vi "Untitled 4.vi"() -> ()   [LabVIEW 2014]
panel:
  in  "Function":enum16{"Init", "Get", "Set", ""}(ring)
  out "data_cluster_out":T1
  in  "data_cluster_in":T1
  out "switch_control_json":string
  out "switch_data_json":string
  out "train_control_json":string
  out "train_data_json":string
  out "train_data_out":T2
  out "switch_control_out":T3
  out "switch_data_out":T4
  out "train_control_out":T5
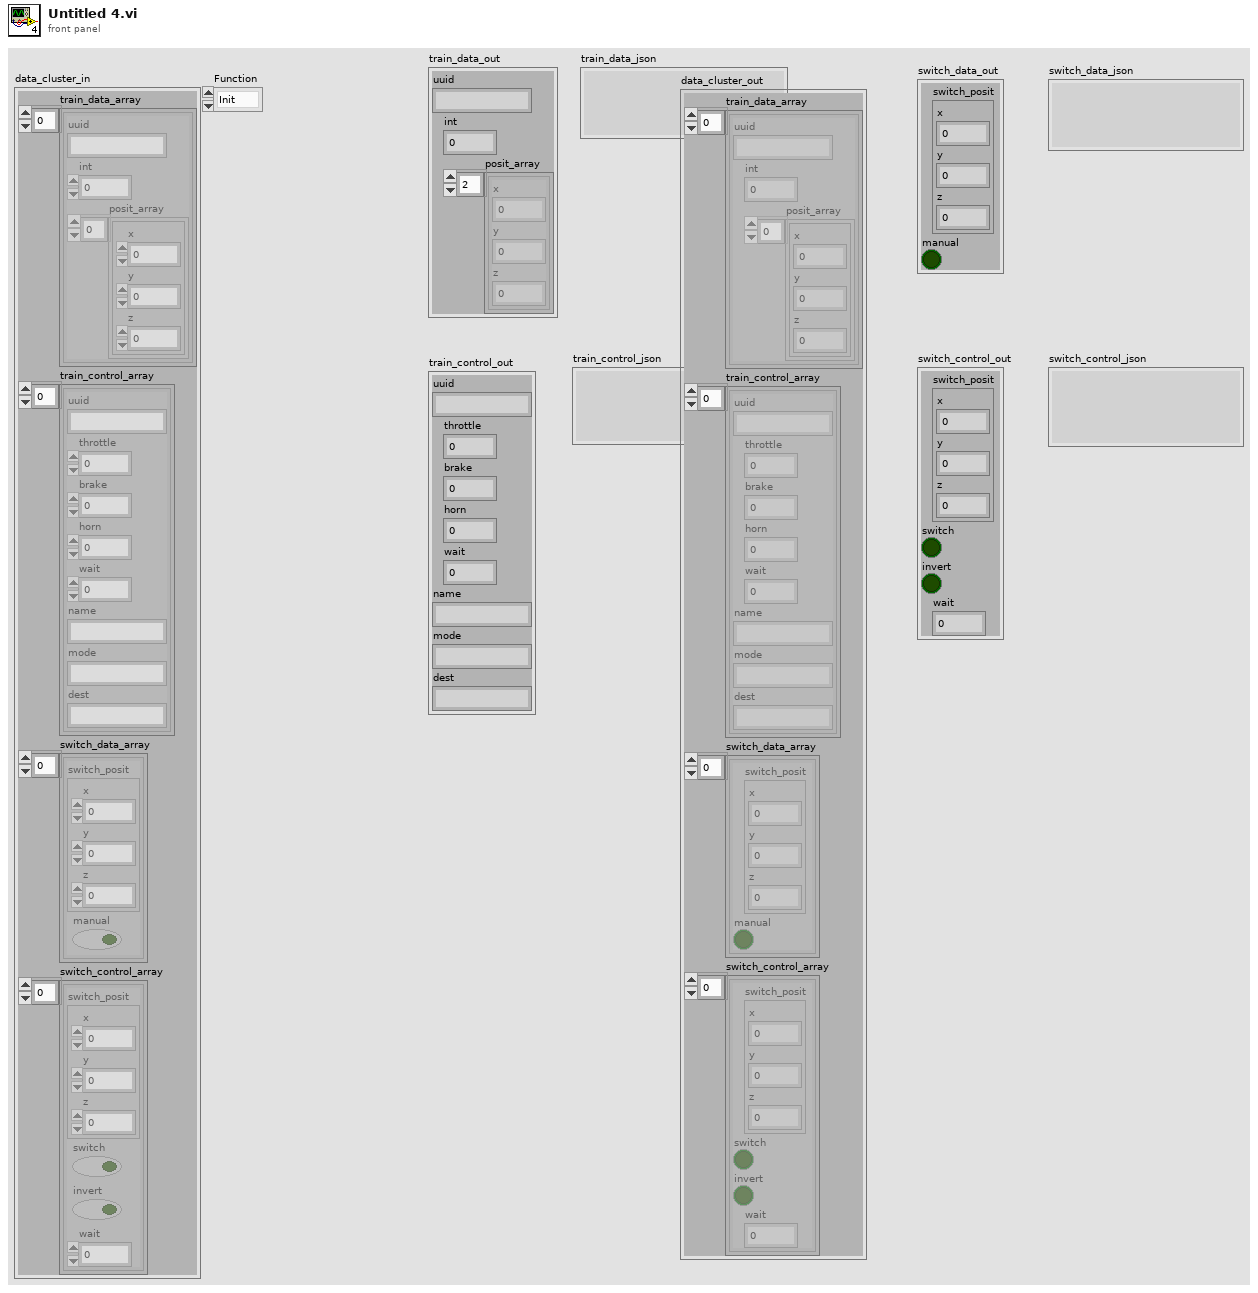
[diagram p1: front panel]
types:
  T1 = cluster{"train_data_array":cluster{"uuid":string, "int":i32, "posit_array":cluster{"x":dbl, "y":dbl, "z":dbl}[]}[], "train_control_array":cluster{"uuid":string, "throttle":dbl, "brake":dbl, "horn":dbl, "wait":dbl, "name":string, "mode":string, "dest":string}[], "switch_data_array":cluster{"switch_posit":cluster{"x":dbl, "y":dbl, "z":dbl}, "manual":bool}[], "switch_control_array":cluster{"switch_posit":cluster{"x":dbl, "y":dbl, "z":dbl}, "switch":bool, "invert":bool, "wait":dbl}[]}
  T2 = cluster{"uuid":string, "int":i32, "posit_array":cluster{"x":dbl, "y":dbl, "z":dbl}[]}
  T3 = cluster{"switch_posit":cluster{"x":dbl, "y":dbl, "z":dbl}, "switch":bool, "invert":bool, "wait":dbl}
  T4 = cluster{"switch_posit":cluster{"x":dbl, "y":dbl, "z":dbl}, "manual":bool}
  T5 = cluster{"uuid":string, "throttle":dbl, "brake":dbl, "horn":dbl, "wait":dbl, "name":string, "mode":string, "dest":string}
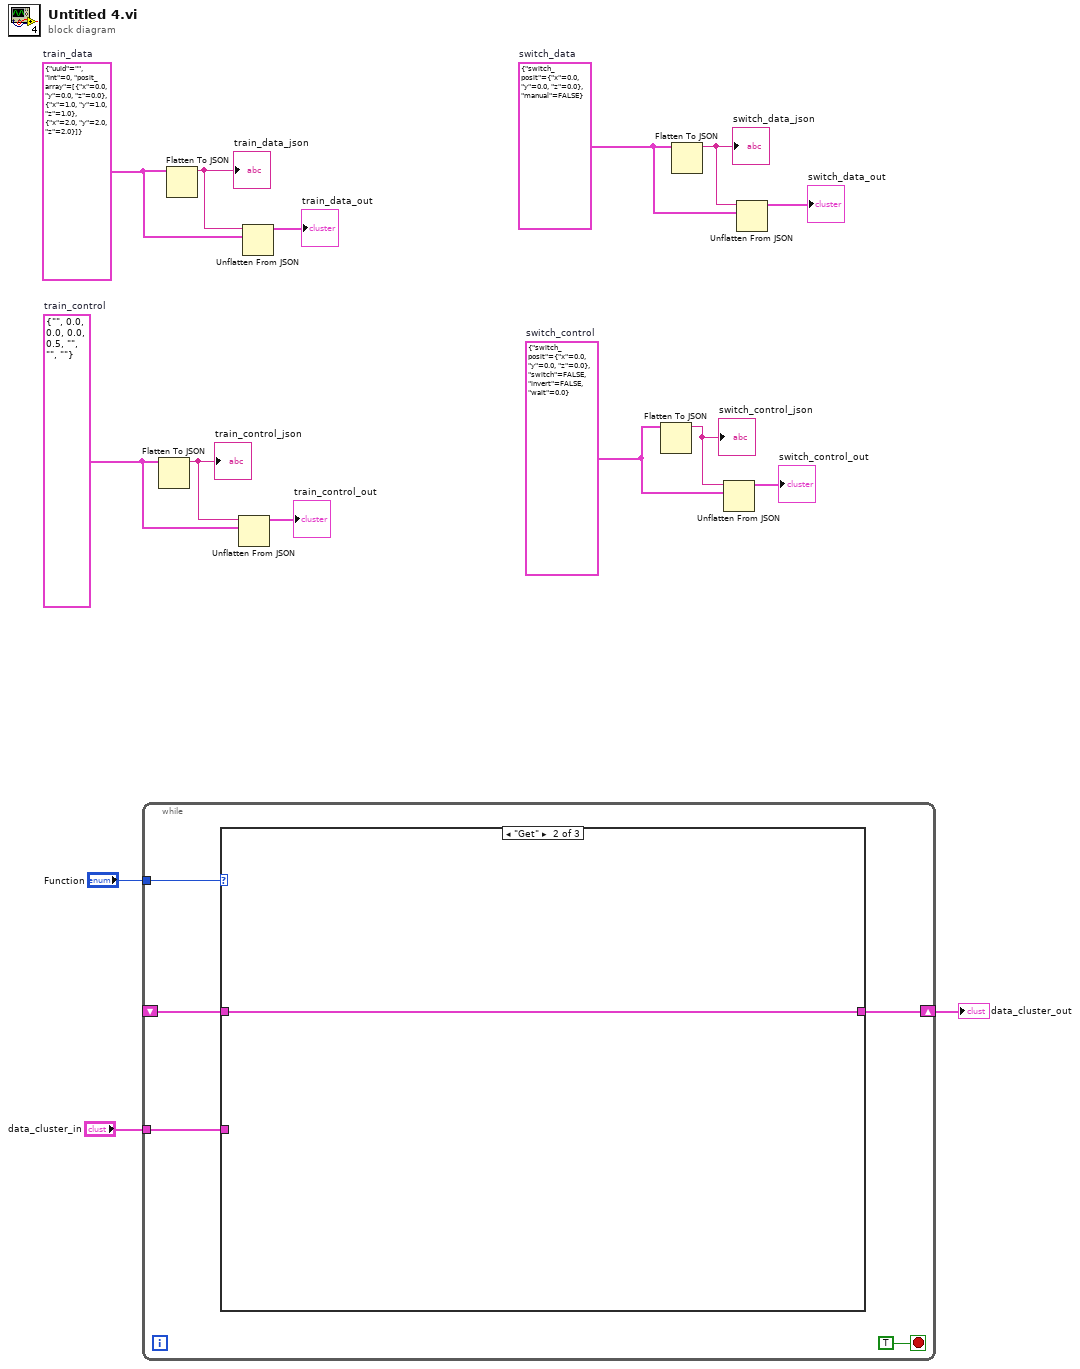
[diagram p0: block diagram]
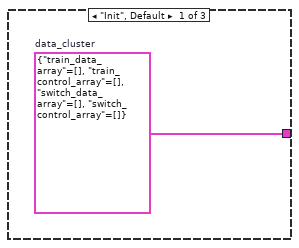
[diagram p2: hidden frame]
diagram:
  w15 = T2 {"uuid"="", "int"=0, "posit_array"=[{"x"=0.0, "y"=0.0, "z"=0.0}, {"x"=1.0, "y"=1.0, "z"=1.0}, {"x"=2.0, "y"=2.0, "z"=2.0}]}  # train_data
  w8 = T3 {"switch_posit"={"x"=0.0, "y"=0.0, "z"=0.0}, "switch"=FALSE, "invert"=FALSE, "wait"=0.0}  # switch_control
  w7 = T4 {"switch_posit"={"x"=0.0, "y"=0.0, "z"=0.0}, "manual"=FALSE}  # switch_data
  w12 = T5 {"uuid"="", "throttle"=0.0, "brake"=0.0, "horn"=0.0, "wait"=0.5, "name"="", "mode"="", "dest"=""}  # train_control
  n1 = while {
    shift-right: [w19] -> w2
    shift-left: _ -> [w18]
    tunnel: "Function" -> [w17]
    tunnel: "data_cluster_in" -> [w16]
    stop <- TRUE stop-if-true
    n2 = case shown="\"Get\"" w17 {
      tunnel: [w21 w22 w23] -> w19
      tunnel: w18 -> [_ w22 _]
      tunnel: w16 -> [_ _ w23]
      frame "Init", Default {
        w21 = T1 {"train_data_array"=[], "train_control_array"=[], "switch_data_array"=[], "switch_control_array"=[]}  # data_cluster
      }
      frame "Get" {
      }
      frame "Set" {
      }
    }
  }
  "data_cluster_out" <- w2
  n3 = Flatten To JSON(anything=w12) -> (JSON string=w13:string)  [unwired: 2 in, 1 out]
  "train_control_json" <- w13
  n4 = Flatten To JSON(anything=w15) -> (JSON string=w14:string)  [unwired: 2 in, 1 out]
  "train_data_json" <- w14
  n5 = Unflatten From JSON(JSON string=w13, type and defaults=w12) -> (value=→"train_control_out":T5)  [unwired: 5 in, 1 out]
  n6 = Unflatten From JSON(JSON string=w14, type and defaults=w15) -> (value=→"train_data_out":T2)  [unwired: 5 in, 1 out]
  n7 = Flatten To JSON(anything=w8) -> (JSON string=w9:string)  [unwired: 2 in, 1 out]
  "switch_control_json" <- w9
  n8 = Flatten To JSON(anything=w7) -> (JSON string=w10:string)  [unwired: 2 in, 1 out]
  "switch_data_json" <- w10
  n9 = Unflatten From JSON(JSON string=w9, type and defaults=w8) -> (value=→"switch_control_out":T3)  [unwired: 5 in, 1 out]
  n10 = Unflatten From JSON(JSON string=w10, type and defaults=w7) -> (value=→"switch_data_out":T4)  [unwired: 5 in, 1 out]
